vi "WPI_CompressorOpen.vi"(0 "Pneumatics Control Module (0)":u8, 11 "error in (no error)":errorcluster) -> (4 "CompressorDevRef":T1, 15 "error out":errorcluster)   [LabVIEW 2017]
doc: "Opens a reference to the compressor you define. You must open a reference before using any other VIs on this palette. After you open a reference to the compressor, you can use the Start and Stop VIs to enable and disable the compressor monitoring and control.\n\nThis software is licensed. Open the labview\\readme\\WPI Robotics Library Open Source License.txt file for more information."
uses:
  <vilib>/Rock Robotics/WPI/Compressor/WPI_CompressorDevRef.ctl
  <vilib>/Rock Robotics/SystemInterfaces/NetworkCommunication/NetComm_UsageReport_ResourceType.ctl
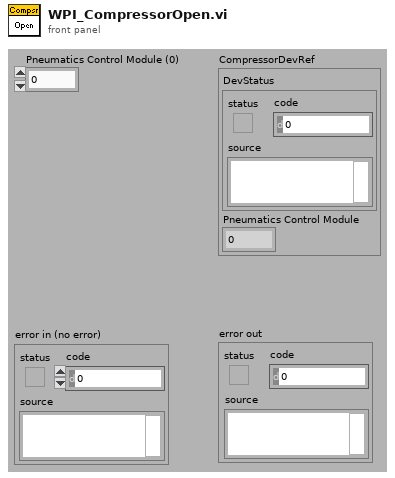
[diagram p1: front panel]
types:
  T1 = typedef "WPI_CompressorDevRef.ctl" = cluster{"DevStatus":errorcluster, "Pneumatics Control Module":u8}
  T2 = typedef "NetComm_UsageReport_ResourceType.ctl" = enum8{"Controller", "Module", "Language", "CANPlugin", "Accelerometer", "ADXL345", "AnalogChannel", "AnalogTrigger", "AnalogTriggerOutput", "CANJaguar", "Compressor", "Counter", "Dashboard", "DigitalInput", "DigitalOutput", "DriverStationCIO", "DriverStationEIO", "DriverStationLCD", "Encoder", "GearTooth", "Gyro", "I2C", "Framework", "Jaguar", "Joystick", "Kinect", "KinectStick", "PIDController", "Preferences", "PWM", "Relay", "RobotDrive", "SerialPort", "Servo", "Solenoid", "SPI", "Task", "Ultrasonic", "Victor", "Button", "Command", "AxisCamera", "PCVideoServer", "SmartDashboard", "Talon", "HiTechnicColorSensor", "HiTechnicAccel", "HiTechnicCompass", "SRF08", "AnalogOutput", "Victor SP", "Talon SRX", "CAN Talon SRX", "ADXL362 Accel", "ADXRS450 Gyro", "Rev SPARK", "Mindsensors SD540", "Digital Filter", "ADIS16448", "PDP", "PCM", "PigeonIMU", "Nidec Brushless", "CTRE CANifier", "CTRE Future 0", "CTRE Future 1", "CTRE Future 2", "CTRE Future 3", "CTRE Future 4", "CTRE Future 5", "CTRE Future 6"}
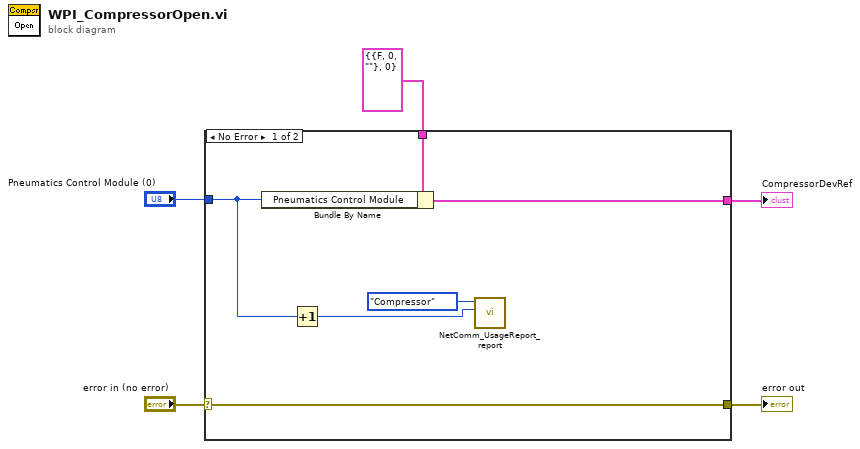
[diagram p0: block diagram]
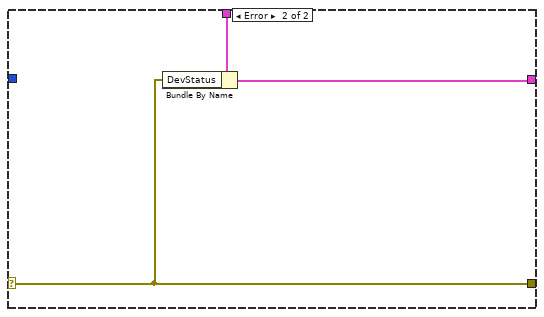
[diagram p2: hidden frame]
diagram:
  n1 = case shown="No Error" "error in (no error)" {
    selector: "error in (no error)" -> [w8 w12]
    tunnel: [w8 w12] -> w5
    tunnel: T1 {"DevStatus"={"status"=FALSE, "code"=0, "source"=""}, "Pneumatics Control Module"=0} ("CompressorDevRef") -> [w11 w14]
    tunnel: [w10 w13] -> w2
    tunnel: "Pneumatics Control Module (0)" -> [w7 _]
    frame No Error {
      n2 = Bundle By Name(cluster=w11, "Pneumatics Control Module"=w7) -> (w10:T1)
      n3 = Increment(x=w7) -> (x+1=w6:u8)
      n4 = call <vilib>:"NetComm_UsageReport_report.vi"("Instance Number"=w6, "Resource Type"=NetComm_UsageReport_ResourceType."Compressor") -> ()  [unwired: 10 in]
    }
    frame Error {
      n5 = Bundle By Name(cluster=w14, "DevStatus"=w12) -> (w13:T1)
    }
  }
  "error out" <- w5
  "CompressorDevRef" <- w2
